vi "Agilent 3352X Series Frequency Sweep.vi"() -> ()   [LabVIEW 2010, in "AWG.lvlib"]
doc: "This example shows how to configure and enable a frequency sweep."
uses:
  AWG.lvlib
  Agilent 3352X Series.lvlib
panel:
  in  "Sweep Time (1 s)":dbl=1.0
  in  "Start Frequency (100 Hz)":dbl=100.0
  in  "Stop  Frequency (1000 Hz)":dbl=1000.0
  in  "Amplitude (0.1 Vpp)":dbl=0.1
  in  "Waveform Function (0: Sine)":u16(ring) items=["Sine"=0, "Square"=1, "Ramp"=2, "Triangle"=5]
  in  "VISA resource name":refnum<visa-resource-name>
  # "(c) 2011-2015 National Instruments.  ALL RIGHTS RESERVED."
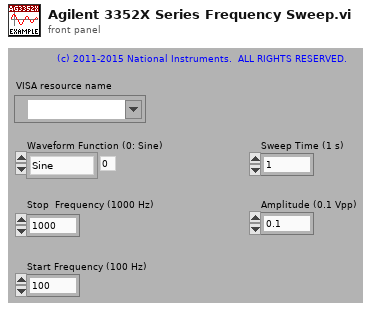
[diagram p1: front panel]
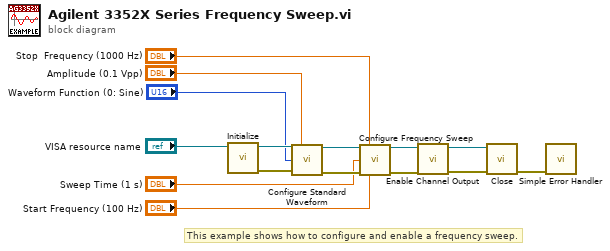
[diagram p0: block diagram]
diagram:
  # "This example shows how to configure and enable a frequency sweep."
  n1 = call "Initialize.vi"("VISA resource name"="VISA resource name") -> ("error out"=w10:errorcluster, "VISA resource name out"=w11:refnum<visa-resource-name>)  [unwired: 4 in, 5 out]
  n2 = call "Configure Standard Waveform.vi"("VISA resource name"=w11, "Amplitude (0.1 Vpp)"="Amplitude (0.1 Vpp)", "Waveform Function (0: Sine)"="Waveform Function (0: Sine)", "error in (no error)"=w10) -> ("VISA resource name out"=w9:refnum<visa-resource-name>, "error out"=w6:errorcluster)  [unwired: 6 in, 4 out]
  n3 = call "Configure Frequency Sweep.vi"("VISA resource name"=w9, "Stop  Frequency (1000 Hz)"="Stop  Frequency (1000 Hz)", "Sweep Time (1 s)"="Sweep Time (1 s)", "error in (no error)"=w6, "Start Frequency (100 Hz)"="Start Frequency (100 Hz)") -> ("VISA resource name out"=w8:refnum<visa-resource-name>, "error out"=w7:errorcluster)  [unwired: 4 in, 5 out]
  n4 = call "Enable Channel Output.vi"("error in (no error)"=w7, "VISA resource name"=w8) -> ("error out"=w13:errorcluster, "VISA resource name out"=w12:refnum<visa-resource-name>)  [unwired: 3 in, 5 out]
  n5 = call "Close.vi"("error in (no error)"=w13, "VISA resource name"=w12) -> ("error out"=w15:errorcluster)  [unwired: 9 out]
  n6 = call <vilib>:"Simple Error Handler.vi"("error in (no error)"=w15) -> ()  [unwired: 1 in, 8 out]
